vi "Get Class Data File Path.vi"() -> (3 "Class Data File Path":path)   [LabVIEW 2020]
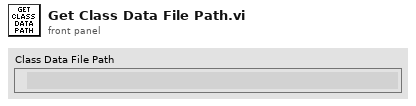
[diagram p1: front panel]
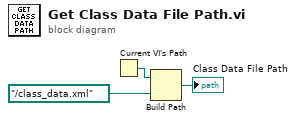
[diagram p0: block diagram]
diagram:
  n1 = Current VI's Path() -> (path=w2:path)
  n2 = Build Path(base path=w2, name or relative path=path "../class_data.xml") -> (appended path=→"Class Data File Path":path)
